vi "ezAFM Practice 1.6.vi"() -> ()   [LabVIEW 2015]
uses:
  D:/LabVIEW for ezAFM/LV-PGC 2019-05a/Special Equipment/ezAFM/NMI Integration Code/ezCommander.dll
  LabVIEW for ezAFM/LV-PGC 2019-05a/Special Equipment/ezAFM/NMI Integration Code/ezCommander.dll
  LabVIEW for ezAFM/LV-PGC 2019-05a/Universal vi's/Global Variables/Globals-EasyAFM.vi
  Globals.vi
  <vilib>/vision/driver/NI_Vision_Acquisition_Software.lvlib
  <vilib>/userdefined/High Color/IMAQdx.ctl
panel:
  out "Test":bool
  out "Index":dbl
  out "Direction":dbl
  out "Searching":bool
  out "Crosshair Found?":bool
  in  "Search":bool
  out "Total Steps":dbl
  out "Current Steps":dbl
  in  "Camera":enum32{"ezAFM Camera"}(tab)
  out "ezAFM Camera":T1(plugin-control)
  in  "Connection to Scan":string
  in  "Enable Automatic \nRepositioning":bool
  out "Imaging Status":string
  out "Automated Imaging":bool
  in  "Main Menu":enum32{"Navigation", "Scanning"}(tab)
  in  "APPROACH":bool
  in  "RETRACT":bool
  in  "Step Size":dbl
  in  "Angle":dbl
  in  "THETA":bool
  in  "MOVE2CROSSHAIR":bool
  in  "Current Crosshair":string(combo)="00 | 01"
  in  "Target Crosshair":string(combo)="00 | 01"
  in  "Motor Speed":u16(ring)=30000 items=["SLOW"=3300, "MEDIUM"=30000, "FAST"=65000]
  in  "Navigation Buttons":T2
  in  "SEARCH":bool
  in  "Image Resolution":u16(ring)=256 items=["32"=32, "64"=64, "128"=128, "256"=256, "512"=512, "1024"=1024, "2048"=2048]
  in  "SELECT CONNECTIONS":bool
  in  "Initialize Automated Imaging":bool
  out "Connections":string[](array[string])
  out "Sequence":string[](array[string])
  in  "Indicators":enum32{"Indicators"}(tab)
  out "XYZ Motor Position":dbl[](array[numeric]) format="%#_4f"
  out "ezAFM Status":dbl
  out "Approaching":bool
  out "ezAFM Connected":bool
  out "Retracting":bool
  out "Scan":bool caption="Scanning"
  out "Tip Approached?":bool
  in  "RESET":bool
  out "XY Position":dbl[](array[numeric])
  in  "QUIT":bool
  # "Use Arrow Keys to manually\nmove the XY Motor"
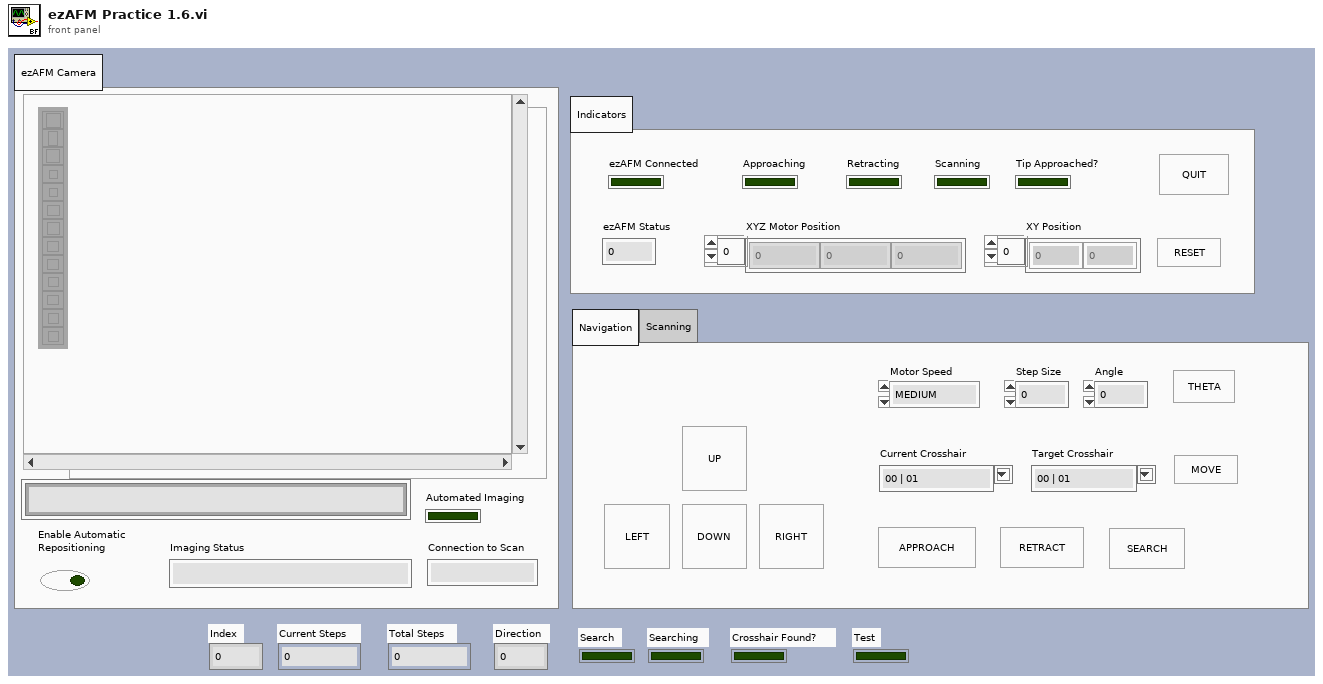
[diagram p1: front panel]
types:
  T1 = typedef "IMAQ Image.ctl" = refnum<image>
  T2 = cluster{"UP":bool, "DOWN":bool, "LEFT":bool, "RIGHT":bool}
  T3 = typedef "IMAQdx.ctl" = refnum<k21>
  T4 = typedef "Image Type" = u32
  T5 = typedef "eventvkey.ctl" = enum16{"ASCII", "Enter", "Return", "Shift", "Ctrl", "Alt", "Cmd", "Opt", "Caps", "NumLock", "Clear", "Break", "Up", "Down", "Left", "Right", "Insert", "Delete", "Home", "End", "PageUp", "PageDown", "Escape", "Help", "Pause", "ScrollLock", "F1", "F2", "F3", "F4", "F5", "F6", "F7", "F8", "F9", "F10", "F11", "F12", "F13", "F14", "F15", "F16", "F17", "F18", "F19", "F20", "F21", "F22", "F23", "F24", "Play", "VolumeUp", "VolumeDown", "Mute", "Two Byte Char"}
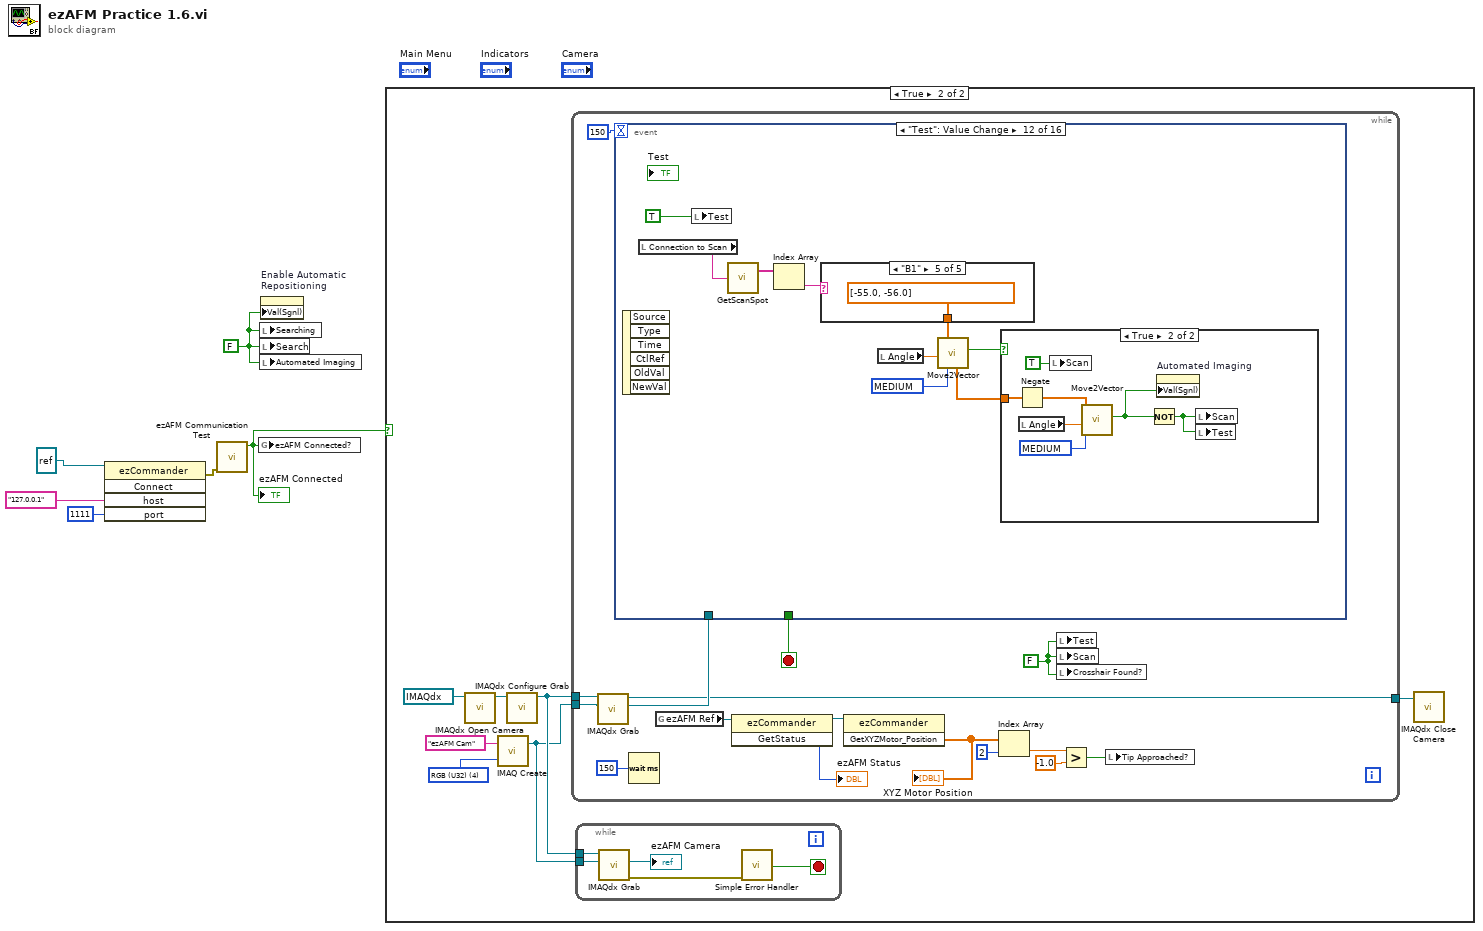
[diagram p0: block diagram]
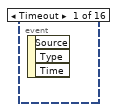
[diagram p3: hidden frame]
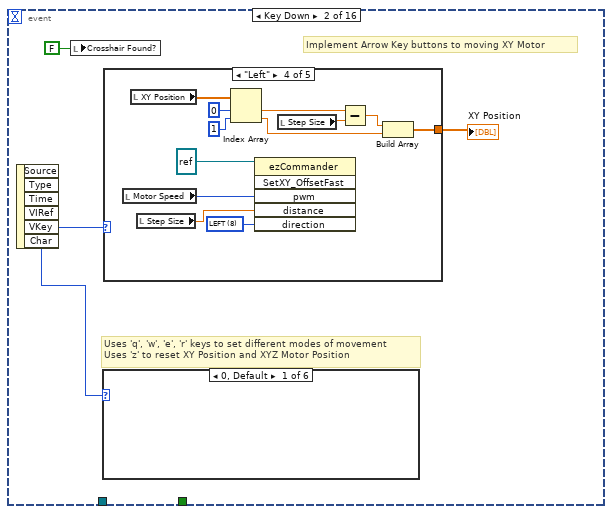
[diagram p4: hidden frame]
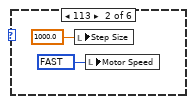
[diagram p5: hidden frame]
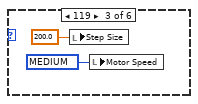
[diagram p6: hidden frame]
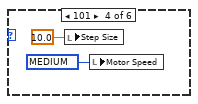
[diagram p7: hidden frame]
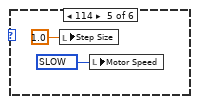
[diagram p8: hidden frame]
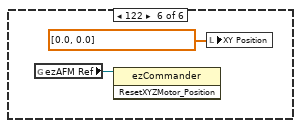
[diagram p9: hidden frame]
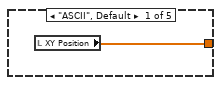
[diagram p10: hidden frame]
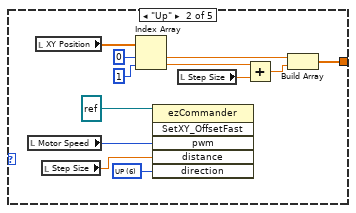
[diagram p11: hidden frame]
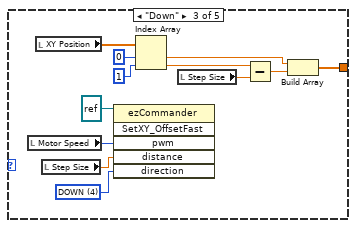
[diagram p12: hidden frame]
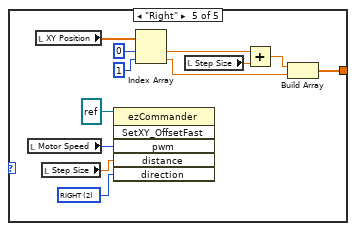
[diagram p13: hidden frame]
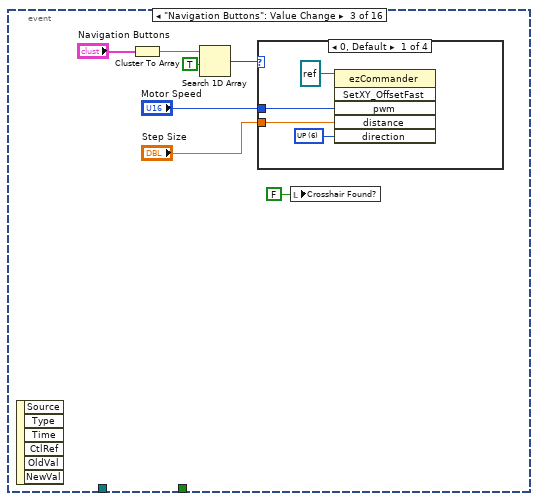
[diagram p14: hidden frame]
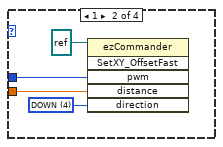
[diagram p15: hidden frame]
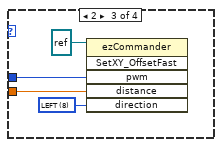
[diagram p16: hidden frame]
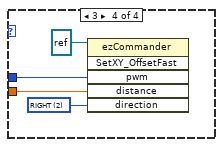
[diagram p17: hidden frame]
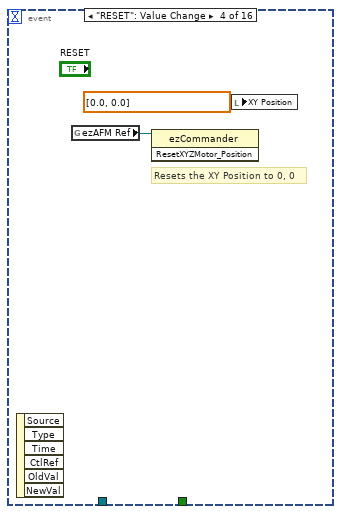
[diagram p18: hidden frame]
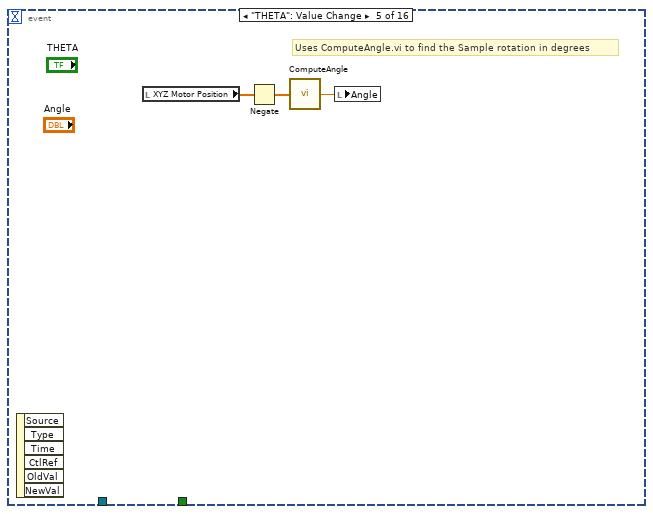
[diagram p19: hidden frame]
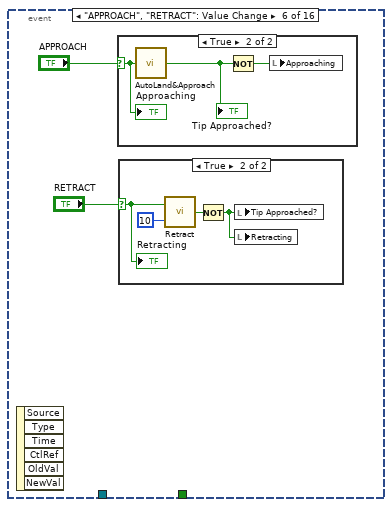
[diagram p20: hidden frame]
diagram:
  w1 = FALSE ("Automated Imaging")
  n1 = invoke class="ezCommander" method="Connect"(reference=refnum<k24> refnum ("ezAFM Ref"), "host"="127.0.0.1", "port"=1111) -> (error out=w5:errorcluster)  [unwired: 2 in, 4 out]
  n2 = call "ezAFM Communication Test.vi"("error in"=w5) -> ("ezAFM COM status"=w2:bool)  [unwired: 3 in, 3 out]
  "ezAFM Connected" <- w2
  n3 = global write "Globals.vi" "ezAFM Connected?"(w2) -> ()
  n4 = local write "Searching"(w1) -> ()
  n5 = local write "Search"(w1) -> ()
  n6 = local write "Automated Imaging"(w1) -> ()
  n7 = property on="Enable Automatic \nRepositioning" class="Bool (strict)"("Val(Sgnl)"=w1) -> ()  [unwired: 2 in, 2 out]
  n8 = case shown="True" w2 {
    frame False {
    }
    frame True {
      w10 = T4 4 items=["Grayscale (U8)", "Grayscale (I16)", "Grayscale (SGL)", "Complex (CSG)", "RGB (U32)", "HSL (U32)", "RGB (U64)", "Grayscale (U16)"] ("Image Type")
      n9 = call <vilib>:"IMAQdx Open Camera.vi"("Session In"=T3 "cam5") -> ("Session Out"=w11:T3)  [unwired: 9 in, 1 out]
      n10 = call "IMAQ Create"("Image Name"="ezAFM Cam", "Image Type"=w10) -> ("New Image"=w8:T1)  [unwired: 3 in, 1 out]
      n11 = call <vilib>:"IMAQdx Configure Grab.vi"("Session In"=w11) -> ("Session Out"=w9:T3)  [unwired: 9 in, 1 out]
      n12 = while {
        tunnel: w9 -> [w24]
        tunnel: w8 -> [w23]
        tunnel: [w21] -> w7
        stop <- w20 stop-if-true
        w19 = FALSE ("Scan")
        n13 = call <vilib>:"IMAQdx Grab.vi"("Image In"=w23, "Session In"=w24) -> ("Image Out"=w22:T1, "Session Out"=w21:T3)  [unwired: 2 in, 6 out]
        n14 = event shown="[11] \"Test\": Value Change" {
          selector: _ -> [_ _ _ _ _ _ _ _ _ _ _ _ _ _ _ _]
          dyn-events: _ -> [_ _ _ _ _ _ _ _ _ _ _ _ _ _ _ _]
          timeout: 150 -> [_ _ _ _ _ _ _ _ _ _ _ _ _ _ _ _]
          tunnel: [_ _ _ _ _ _ _ _ _ _ _ _ _ _ _ "QUIT"] -> w20
          tunnel: w22 -> [_ _ _ _ _ _ _ _ _ _ _ _ _ w207 _ _]
          event Timeout {
            n15 = event-data() -> ()  [unwired: 1 in, 3 out]
          }
          event Key Down {
            # "Uses 'q', 'w', 'e', 'r' keys to set different modes of movement\nUses 'z' to reset XY Position and XYZ Motor Position"
            # "Implement Arrow Key buttons to moving XY Motor"
            n16 = event-data() -> ("VKey"=w36:T5, "Char"=w37:i16)  [unwired: 1 in, 4 out]
            n17 = local write "Crosshair Found?"(FALSE ("Crosshair Found?")) -> ()
            n18 = case shown="0, Default" w37 {
              frame 0, Default {
              }
              frame 113 {
                w39 = u16 65000 items=["SLOW"=3300, "MEDIUM"=30000, "FAST"=65000] ("Motor Speed")
                n19 = local write "Step Size"(1000.0 ("Step Size")) -> ()
                n20 = local write "Motor Speed"(w39) -> ()
              }
              frame 119 {
                w41 = u16 30000 items=["SLOW"=3300, "MEDIUM"=30000, "FAST"=65000] ("Motor Speed")
                n21 = local write "Step Size"(200.0 ("Step Size")) -> ()
                n22 = local write "Motor Speed"(w41) -> ()
              }
              frame 101 {
                w43 = u16 30000 items=["SLOW"=3300, "MEDIUM"=30000, "FAST"=65000] ("Motor Speed")
                n23 = local write "Step Size"(10.0 ("Step Size")) -> ()
                n24 = local write "Motor Speed"(w43) -> ()
              }
              frame 114 {
                w45 = u16 3300 items=["SLOW"=3300, "MEDIUM"=30000, "FAST"=65000] ("Motor Speed")
                n25 = local write "Step Size"(1.0 ("Step Size")) -> ()
                n26 = local write "Motor Speed"(w45) -> ()
              }
              frame 122 {
                n27 = global read "Globals-EasyAFM.vi" "ezAFM Ref"() -> (w47:refnum<k24>)
                n28 = invoke class="ezCommander" method="ResetXYZMotor_Position"(reference=w47) -> ()  [unwired: 2 in, 3 out]
                n29 = local write "XY Position"(dbl[] [0.0, 0.0] ("XY Position")) -> ()
              }
            }
            n30 = case shown="\"Left\"" w36 {
              tunnel: [w49 w51 w62 w74 w86] -> w38
              frame "ASCII", Default {
                n31 = local read "XY Position"() -> (w49:dbl[])
              }
              frame "Up" {
                w60 = u16 6 items=["UP"=6, "DOWN"=4, "LEFT"=8, "RIGHT"=2]
                n32 = local read "Motor Speed"() -> (w59:u16)
                n33 = local read "XY Position"() -> (w57:dbl[])
                n34 = local read "Step Size"() -> (w58:dbl)
                n35 = Index Array(array=w57, index #1=0 ("index"), index #2=1 ("index")) -> (element #1=w53:dbl, element #2=w50:dbl)
                n36 = invoke class="ezCommander" method="SetXY_OffsetFast"(reference=refnum<k24> refnum ("ezAFM Ref"), "pwm"=w59, "distance"=w58, "direction"=w60) -> ()  [unwired: 2 in, 6 out]
                n37 = local read "Step Size"() -> (w54:dbl)
                n38 = Add(x=w50, y=w54) -> (x+y=w52:dbl)
                n39 = Build Array(w53, w52) -> (w51:dbl[])
              }
              frame "Down" {
                w70 = u16 4 items=["UP"=6, "DOWN"=4, "LEFT"=8, "RIGHT"=2]
                n40 = local read "Motor Speed"() -> (w72:u16)
                n41 = local read "XY Position"() -> (w64:dbl[])
                n42 = local read "Step Size"() -> (w71:dbl)
                n43 = invoke class="ezCommander" method="SetXY_OffsetFast"(reference=refnum<k24> refnum ("ezAFM Ref"), "pwm"=w72, "distance"=w71, "direction"=w70) -> ()  [unwired: 2 in, 6 out]
                n44 = Index Array(array=w64, index #1=0 ("index"), index #2=1 ("index")) -> (element #1=w66:dbl, element #2=w67:dbl)
                n45 = local read "Step Size"() -> (w63:dbl)
                n46 = Subtract(x=w67, y=w63) -> (x-y=w65:dbl)
                n47 = Build Array(w66, w65) -> (w62:dbl[])
              }
              frame "Left" {
                w84 = u16 8 items=["UP"=6, "DOWN"=4, "LEFT"=8, "RIGHT"=2]
                n48 = local read "Motor Speed"() -> (w82:u16)
                n49 = local read "XY Position"() -> (w78:dbl[])
                n50 = local read "Step Size"() -> (w83:dbl)
                n51 = Index Array(array=w78, index #1=0 ("index"), index #2=1 ("index")) -> (element #1=w77:dbl, element #2=w75:dbl)
                n52 = invoke class="ezCommander" method="SetXY_OffsetFast"(reference=refnum<k24> refnum ("ezAFM Ref"), "pwm"=w82, "distance"=w83, "direction"=w84) -> ()  [unwired: 2 in, 6 out]
                n53 = local read "Step Size"() -> (w79:dbl)
                n54 = Subtract(x=w77, y=w79) -> (x-y=w76:dbl)
                n55 = Build Array(w76, w75) -> (w74:dbl[])
              }
              frame "Right" {
                w96 = u16 2 items=["UP"=6, "DOWN"=4, "LEFT"=8, "RIGHT"=2]
                n56 = local read "Motor Speed"() -> (w95:u16)
                n57 = local read "XY Position"() -> (w91:dbl[])
                n58 = local read "Step Size"() -> (w94:dbl)
                n59 = invoke class="ezCommander" method="SetXY_OffsetFast"(reference=refnum<k24> refnum ("ezAFM Ref"), "pwm"=w95, "distance"=w94, "direction"=w96) -> ()  [unwired: 2 in, 6 out]
                n60 = Index Array(array=w91, index #1=0 ("index"), index #2=1 ("index")) -> (element #1=w89:dbl, element #2=w87:dbl)
                n61 = local read "Step Size"() -> (w90:dbl)
                n62 = Add(x=w89, y=w90) -> (x+y=w88:dbl)
                n63 = Build Array(w88, w87) -> (w86:dbl[])
              }
            }
            "XY Position" <- w38
          }
          event "Navigation Buttons": Value Change {
            n64 = event-data() -> ()  [unwired: 1 in, 6 out]
            n65 = Cluster To Array(cluster="Navigation Buttons") -> (array=w103:bool[])
            n66 = Search 1D Array(1D array=w103, element=TRUE) -> (index of element=w101:i32)  [unwired: 1 in]
            n67 = case shown="0, Default" w101 {
              tunnel: "Step Size" -> [w105 w110 w114 w118]
              tunnel: "Motor Speed" -> [w106 w109 w113 w117]
              frame 0, Default {
                w107 = u16 6 items=["UP"=6, "DOWN"=4, "LEFT"=8, "RIGHT"=2]
                n68 = invoke class="ezCommander" method="SetXY_OffsetFast"(reference=refnum<k24> refnum ("ezAFM Ref"), "pwm"=w106, "distance"=w105, "direction"=w107) -> ()  [unwired: 2 in, 6 out]
              }
              frame 1 {
                w111 = u16 4 items=["UP"=6, "DOWN"=4, "LEFT"=8, "RIGHT"=2]
                n69 = invoke class="ezCommander" method="SetXY_OffsetFast"(reference=refnum<k24> refnum ("ezAFM Ref"), "pwm"=w109, "distance"=w110, "direction"=w111) -> ()  [unwired: 2 in, 6 out]
              }
              frame 2 {
                w115 = u16 8 items=["UP"=6, "DOWN"=4, "LEFT"=8, "RIGHT"=2]
                n70 = invoke class="ezCommander" method="SetXY_OffsetFast"(reference=refnum<k24> refnum ("ezAFM Ref"), "pwm"=w113, "distance"=w114, "direction"=w115) -> ()  [unwired: 2 in, 6 out]
              }
              frame 3 {
                w119 = u16 2 items=["UP"=6, "DOWN"=4, "LEFT"=8, "RIGHT"=2]
                n71 = invoke class="ezCommander" method="SetXY_OffsetFast"(reference=refnum<k24> refnum ("ezAFM Ref"), "pwm"=w117, "distance"=w118, "direction"=w119) -> ()  [unwired: 2 in, 6 out]
              }
            }
            n72 = local write "Crosshair Found?"(FALSE ("Crosshair Found?")) -> ()
          }
          event "RESET": Value Change {
            # "Resets the XY Position to 0, 0"
            n73 = event-data() -> ()  [unwired: 1 in, 6 out]
            n74 = global read "Globals-EasyAFM.vi" "ezAFM Ref"() -> (w121:refnum<k24>)
            n75 = invoke class="ezCommander" method="ResetXYZMotor_Position"(reference=w121) -> ()  [unwired: 2 in, 3 out]
            n76 = local write "XY Position"(dbl[] [0.0, 0.0] ("XY Position")) -> ()
          }
          event "THETA": Value Change {
            # "Uses ComputeAngle.vi to find the Sample rotation in degrees"
            n77 = event-data() -> ()  [unwired: 1 in, 6 out]
            n78 = local read "XYZ Motor Position"() -> (w124:dbl[])
            n79 = Negate(x=w124) -> (-x=w125:dbl[])
            n80 = call "ComputeAngle.vi"("XY Vector"=w125) -> ("Angle"=w123:dbl)
            n81 = local write "Angle"(w123) -> ()
          }
          event "APPROACH", "RETRACT": Value Change {
            n82 = event-data() -> ()  [unwired: 1 in, 6 out]
            n83 = case shown="True" "APPROACH" {
              selector: "APPROACH" -> [_ w133]
              frame False {
              }
              frame True {
                n84 = call "AutoLand&Approach.vi"("Approaching?"=w133) -> ("Finished?"=w132:bool)
                "Tip Approached?" <- w132
                n85 = Not(x=w132) -> (.not. x?=w134:bool)
                n86 = local write "Approaching"(w134) -> ()
                "Approaching" <- w133
              }
            }
            n87 = case shown="True" "RETRACT" {
              selector: "RETRACT" -> [_ w128]
              frame False {
              }
              frame True {
                n88 = call "Retract.vi"("Number of Cycles"=10, "Retracting?"=w128) -> ("Finished?"=w130:bool)
                n89 = Not(x=w130) -> (.not. x?=w129:bool)
                n90 = local write "Tip Approached?"(w129) -> ()
                n91 = local write "Retracting"(w129) -> ()
                "Retracting" <- w128
              }
            }
          }
          event "MOVE2CROSSHAIR": Value Change {
            w139 = u16 65000 items=["SLOW"=3300, "MEDIUM"=30000, "FAST"=65000] ("Motor Speed")
            # "XY Vector is in cartesian coordinates of the Oasis Camera\nUses Move2Device.vi to find the XY Vector between the Current Device and Target Device crosshairs\nInputs the XY Vector into Move2Vector.vi to command the XY Motor to move"
            n92 = event-data() -> ()  [unwired: 1 in, 6 out]
            n93 = call "GetDeviceVector.vi"("Target Device"="Target Crosshair", "Current Device"="Current Crosshair") -> ("XY Vector"=w140:dbl[])
            n94 = local read "Angle"() -> (w138:dbl)
            n95 = call "Move2Vector.vi"("Motor Speed"=w139, "Angle"=w138, "XY Vector"=w140) -> ("Finished?"=w135:bool)  [unwired: 8 in]
            n96 = case shown="True" w135 {
              frame False {
              }
              frame True {
                n97 = local read "Enable Automatic \nRepositioning"() -> (w143:bool)
                n98 = local read "Target Crosshair"() -> (w142:string)
                n99 = local write "MOVE2CROSSHAIR"(FALSE) -> ()
                n100 = local write "Current Crosshair"(w142) -> ()
                n101 = case shown="True" w143 {
                  frame False {
                  }
                  frame True {
                    n102 = property on="Search" class="Bool (strict)"("Val(Sgnl)"=TRUE ("Value (Signaling)")) -> ()  [unwired: 2 in, 2 out]
                  }
                }
              }
            }
          }
          event "SELECT CONNECTIONS": Value Change {
            n103 = event-data() -> ()  [unwired: 1 in, 6 out]
            n104 = case shown="True" "SELECT CONNECTIONS" {
              frame False {
              }
              frame True {
                n105 = call "SelectConnections.vi"() -> ("Selected Connections"=→"Connections":string[])  [unwired: 1 in]
              }
            }
          }
          event "Initialize Automated Imaging": Value Change {
            n106 = event-data() -> ()  [unwired: 1 in, 6 out]
            n107 = local read "Connections"() -> (w151:string[])
            n108 = call "BuildSequence.vi"("Connections"=w151) -> ("Sequence"=w149:string[])
            "Sequence" <- w149
            n109 = Array Size(array=w149) -> (size(s)=w148:i32)
            n110 = Greater Than 0?(x=w148) -> (x > 0?=w147:bool)
            n111 = local write "Enable Automatic \nRepositioning"(w147) -> ()
            n112 = local write "Automated Imaging"(w147) -> ()
            n113 = property on="Automated Imaging" class="Bool (strict)"("Val(Sgnl)"=w147) -> ()  [unwired: 2 in, 2 out]
            "Index" <- -1.0 ("Index")
          }
          event "Automated Imaging": Value Change {
            n114 = event-data() -> ()  [unwired: 1 in, 6 out]
            n115 = local read "Index"() -> (w156:dbl)
            n116 = local read "Sequence"() -> (w154:string[])
            n117 = Increment(x=w156) -> (x+1=w155:dbl)
            n118 = local write "Index"(w155) -> ()
            n119 = Index Array(array=w154, index=w155) -> (element=w153:string)
            "Imaging Status" <- w153
            n120 = Search/Split String(string=w153, search string/char (-)="Scan Spot") -> (offset of match=w159:i32)  [unwired: 1 in, 2 out]
            n121 = Search/Split String(string=w153, search string/char (-)="Crosshairs") -> (offset of match=w160:i32)  [unwired: 1 in, 2 out]
            n122 = Greater Or Equal To 0?(x=w159) -> (x >= 0?=w158:bool)
            n123 = Greater Or Equal To 0?(x=w160) -> (x >= 0?=w157:bool)
            n124 = case shown="True" w157 {
              tunnel: w153 -> [_ w170]
              frame False {
              }
              frame True {
                n125 = String Subset(string=w170, offset (0)=21, length (rest)=7 ("length (rest)")) -> (substring=w164:string)
                n126 = String Subset(string=w170, offset (0)=10, length (rest)=7 ("length (rest)")) -> (substring=w165:string)
                n127 = local write "Current Crosshair"(w165) -> ()
                n128 = local write "Target Crosshair"(w164) -> ()
                n129 = String Length(string=w165) -> (length=w166:i32)
                n130 = String Length(string=w164) -> (length=w167:i32)
                n131 = Greater Than 0?(x=w166) -> (x > 0?=w168:bool)
                n132 = Greater Than 0?(x=w167) -> (x > 0?=w169:bool)
                n133 = And(x=w168, y=w169) -> (x .and. y?=w163:bool)
                n134 = property on="MOVE2CROSSHAIR" class="Bool (strict)"("Val(Sgnl)"=w163) -> ()  [unwired: 2 in, 2 out]
              }
            }
            n135 = case shown="True" w158 {
              tunnel: w153 -> [_ w179]
              frame False {
              }
              frame True {
                n136 = String Subset(string=w179, offset (0)=25) -> (substring=w176:string)  [unwired: 1 in]
                n137 = local write "Connection to Scan"(w176) -> ()
                n138 = String Length(string=w176) -> (length=w177:i32)
                n139 = Greater Than 0?(x=w177) -> (x > 0?=w175:bool)
                n140 = property on="Test" class="Bool (strict)"("Val(Sgnl)"=w175) -> ()  [unwired: 2 in, 2 out]
              }
            }
            n141 = Wait (ms)(milliseconds to wait=u32 1000) -> ()  [unwired: 1 out]
          }
          event "Scan": Value Change {
            n142 = event-data() -> ()  [unwired: 1 in, 6 out]
            n143 = local read "Angle"() -> (w181:dbl)
            n144 = call "TakeScan.vi"("Angle"=w181, "Image Resolution"="Image Resolution", "Connection"="Connection to Scan") -> (1:w180)  [unwired: 7 in, 1 out]
            n145 = local write "Scan"(w180) -> ()
          }
          event "Test": Value Change {
            w188 = u16 30000 items=["SLOW"=3300, "MEDIUM"=30000, "FAST"=65000] ("Motor Speed")
            n146 = event-data() -> ()  [unwired: 1 in, 6 out]
            n147 = local read "Connection to Scan"() -> (w191:string)
            n148 = local write "Test"(TRUE ("Fine Navigation")) -> ()
            n149 = call "GetScanSpot.vi"("Device to Scan"=w191) -> ("Scan Spot"=w190:string[])  [unwired: 1 out]
            n150 = Index Array(array=w190) -> (element=w189:string)  [unwired: 1 in]
            n151 = case shown="\"B1\"" w189 {
              tunnel: [dbl[] [0.0, 0.0] ("XY Vector") dbl[] [-73.0, 35.0] ("XY Vector") dbl[] [-55.0, 35.0] ("XY Vector") dbl[] [-73.0, -56.0] ("XY Vector") dbl[] [-55.0, -56.0] ("XY Vector")] -> w185
              frame "NONE", Default {
              }
              frame "A0" {
              }
              frame "B0" {
              }
              frame "A1" {
              }
              frame "B1" {
              }
            }
            n152 = local read "Angle"() -> (w187:dbl)
            n153 = call "Move2Vector.vi"("Motor Speed"=w188, "Angle"=w187, "XY Vector"=w185) -> ("Finished?"=w186:bool)  [unwired: 8 in]
            n154 = case shown="True" w186 {
              tunnel: w185 -> [_ w195]
              frame False {
              }
              frame True {
                w196 = u16 30000 items=["SLOW"=3300, "MEDIUM"=30000, "FAST"=65000] ("Motor Speed")
                n155 = Negate(x=w195) -> (-x=w194:dbl[])
                n156 = local read "Angle"() -> (w197:dbl)
                n157 = local write "Scan"(TRUE ("Scan")) -> ()
                n158 = call "Move2Vector.vi"("Motor Speed"=w196, "Angle"=w197, "XY Vector"=w194) -> ("Finished?"=w193:bool)  [unwired: 8 in]
                n159 = Not(x=w193) -> (.not. x?=w192:bool)
                n160 = property on="Automated Imaging" class="Bool (strict)"("Val(Sgnl)"=w193) -> ()  [unwired: 2 in, 2 out]
                n161 = local write "Scan"(w192) -> ()
                n162 = local write "Test"(w192) -> ()
              }
            }
          }
          event "Enable Automatic \nRepositioning": Value Change {
            w204 = u16 6 items=["UP"=6, "DOWN"=4, "LEFT"=8, "RIGHT"=2]
            n163 = event-data() -> ()  [unwired: 1 in, 6 out]
            "Total Steps" <- 1.0 ("Total Distance")
            "Current Steps" <- 0.0 ("Current Steps")
            "Direction" <- w204
          }
          event "SEARCH", "Search": Value Change {
            n164 = event-data() -> ("NewVal"=w208:bool)  [unwired: 1 in, 5 out]
            n165 = while {
              tunnel: w207 -> [w217]
              tunnel: [w213] -> w209
              tunnel: [w216] -> w210
              i -> [w214]
              stop <- w211 stop-if-true
              n166 = Greater?(x=w214, y=5.0) -> (0:w212:bool)
              n167 = call "IdentifyCrosshair.vi"("ezAFM Camera"=w217) -> ("Delta"=w216:dbl[], "Found?"=w213:bool)
              n168 = Or(x=w212, y=w213) -> (x .or. y?=w211:bool)
            }
            "Crosshair Found?" <- w209
            n169 = local write "Searching"(w208) -> ()
            n170 = case shown="False" w209 {
              tunnel: w210 -> [_ w228]
              frame False {
                n171 = local read "Enable Automatic \nRepositioning"() -> (w219:bool)
                n172 = local write "Searching"(FALSE ("Searching")) -> ()
                n173 = case shown="True" w219 {
                  frame False {
                  }
                  frame True {
                    n174 = property on="Searching" class="Bool (strict)"("Val(Sgnl)"=TRUE ("Value (Signaling)")) -> ()  [unwired: 2 in, 2 out]
                  }
                }
              }
              frame True {
                w226 = FALSE ("SEARCH")
                w227 = u16 3300 items=["SLOW"=3300, "MEDIUM"=30000, "FAST"=65000] ("Motor Speed")
                n175 = local write "Search"(w226) -> ()
                n176 = local write "Searching"(w226) -> ()
                n177 = call "Move2Vector.vi"("Motor Speed"=w227, "Angle"=0.0, "XY Vector"=w228) -> ("Finished?"=w221:bool)  [unwired: 8 in]
                n178 = local read "Automated Imaging"() -> (w223:bool)
                n179 = property on="Enable Automatic \nRepositioning" class="Bool (strict)"("Val(Sgnl)"=TRUE ("Value (Signaling)")) -> ()  [unwired: 2 in, 2 out]
                n180 = And(x=w223, y=w221) -> (x .and. y?=w222:bool)
                n181 = case shown="True" w222 {
                  selector: w222 -> [_ w229]
                  frame False {
                  }
                  frame True {
                    n182 = property on="Automated Imaging" class="Bool (strict)"("Val(Sgnl)"=w229) -> ()  [unwired: 2 in, 2 out]
                  }
                }
              }
            }
          }
          event "Searching": Value Change {
            n183 = event-data() -> ()  [unwired: 1 in, 6 out]
            n184 = local read "Total Steps"() -> (w231:dbl)
            n185 = local read "Current Steps"() -> (w232:dbl)
            n186 = local read "Direction"() -> (w233:dbl)
            n187 = Equal?(x=w231, y=w232) -> (x = y?=w234:bool)
            n188 = case shown="False" w234 {
              tunnel: w232 -> [w238 _]
              tunnel: w233 -> [w239 w246]
              tunnel: w231 -> [_ w245]
              tunnel: [TRUE ("Value (Signaling)") TRUE ("Value (Signaling)")] -> w230
              frame False {
                w240 = u16 30000 items=["SLOW"=3300, "MEDIUM"=30000, "FAST"=65000] ("Motor Speed")
                n189 = Increment(x=w238) -> (x+1=w237:dbl)
                n190 = local write "Current Steps"(w237) -> ()
                n191 = invoke class="ezCommander" method="SetXY_OffsetFast"(reference=refnum<k24> refnum ("ezAFM Ref"), "pwm"=w240, "distance"=20.0, "direction"=w239) -> ()  [unwired: 2 in, 6 out]
                n192 = Wait (ms)(milliseconds to wait=u32 5000) -> ()  [unwired: 1 out]
              }
              frame True {
                n193 = case shown="6" w246 {
                  tunnel: [u16 0 w251 w252 w253 w254] -> w244
                  frame Default {
                  }
                  frame 6 {
                    w251 = u16 2 items=["UP"=6, "DOWN"=4, "LEFT"=8, "RIGHT"=2]
                  }
                  frame 4 {
                    w252 = u16 8 items=["UP"=6, "DOWN"=4, "LEFT"=8, "RIGHT"=2]
                  }
                  frame 8 {
                    w253 = u16 6 items=["UP"=6, "DOWN"=4, "LEFT"=8, "RIGHT"=2]
                  }
                  frame 2 {
                    w254 = u16 4 items=["UP"=6, "DOWN"=4, "LEFT"=8, "RIGHT"=2]
                  }
                }
                n194 = local write "Current Steps"(0.0 ("Current Steps")) -> ()
                n195 = local write "Direction"(w244) -> ()
                n196 = case shown="6" w244 {
                  tunnel: w245 -> [_ w248]
                  frame Default {
                  }
                  frame 6 {
                    n197 = Increment(x=w248) -> (x+1=w249:dbl)
                    n198 = local write "Total Steps"(w249) -> ()
                  }
                }
              }
            }
            n199 = property on="Search" class="Bool (strict)"("Val(Sgnl)"=w230) -> ()  [unwired: 2 in, 2 out]
          }
          event "QUIT": Value Change {
            w256 = FALSE ("ezAFM Connected?")
            n200 = event-data() -> ()  [unwired: 1 in, 6 out]
            n201 = global write "Globals.vi" "ezAFM Connected?"(w256) -> ()
            n202 = local write "ezAFM Connected"(w256) -> ()
          }
        }
        n203 = Wait (ms)(milliseconds to wait=u32 150) -> ()  [unwired: 1 out]
        n204 = global read "Globals-EasyAFM.vi" "ezAFM Ref"() -> (w26:refnum<k24>)
        n205 = invoke class="ezCommander" method="GetStatus"(reference=w26) -> (reference out=w28:refnum<k24>, "GetStatus"=→"ezAFM Status":i32)  [unwired: 2 in, 1 out]
        n206 = invoke class="ezCommander" method="GetXYZMotor_Position"(reference=w28) -> ("GetXYZMotor_Position"=w29:dbl[])  [unwired: 2 in, 2 out]
        "XYZ Motor Position" <- w29
        n207 = Index Array(array=w29, index=2) -> (element=w30:dbl)
        n208 = local write "Test"(w19) -> ()
        n209 = local write "Scan"(w19) -> ()
        n210 = local write "Crosshair Found?"(w19) -> ()
        n211 = Greater?(x=w30, y=-1.0) -> (0:w25:bool)
        n212 = local write "Tip Approached?"(w25) -> ()
      }
      n213 = while {
        tunnel: w9 -> [w18]
        tunnel: w8 -> [w17]
        stop <- w14 stop-if-true
        n214 = call <vilib>:"IMAQdx Grab.vi"("Image In"=w17, "Session In"=w18) -> ("error out"=w15:errorcluster, "Image Out"=→"ezAFM Camera":T1)  [unwired: 2 in, 6 out]
        n215 = call <vilib>:"Simple Error Handler.vi"("error in (no error)"=w15) -> ("error?"=w14:bool)  [unwired: 4 in, 4 out]
      }
      n216 = call <vilib>:"IMAQdx Close Camera.vi"("Session In"=w7) -> ()  [unwired: 10 in, 1 out]
    }
  }
